vi "写校准时间及fid.vi"(8 "error in (no error)":errorcluster, 9 "量程":u16, 10 "fid":u16, 11 "MB session in":refnum<class "MB_Master.lvclass">) -> (0 "error out":errorcluster, 3 "MB session out":refnum<class "MB_Master.lvclass">)   [LabVIEW 2016, in "MB SLAVE.lvlib"]
uses:
  MB SLAVE.lvlib
  <vilib>/Plasmionique/MB Master/MB_Master/MB_Master.lvclass
  <vilib>/Plasmionique/MB Master/MB Master.lvlib
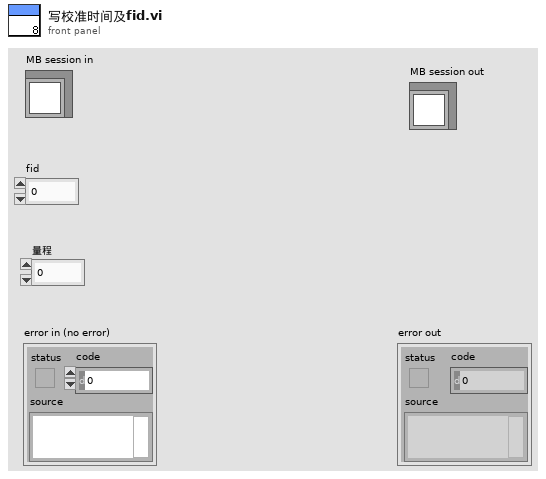
[diagram p1: front panel]
types:
  T1 = typedef "LVDateTimeRec.ctl" = cluster{"秒数的小数部分":dbl, "秒":i32, "分":i32, "时":i32, "日":i32, "月":i32, "年":i32, "天数（周）":i32, "天数（年）":i32, "DST":i32}
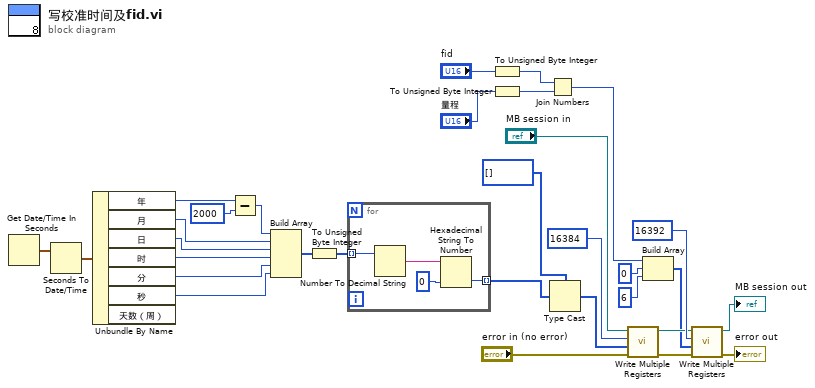
[diagram p0: block diagram]
diagram:
  n1 = Get Date/Time In Seconds() -> (seconds since 1Jan1904=w22:timestamp)
  n2 = Seconds To Date/Time(time stamp (now)=w22) -> (date time rec=w23:T1)  [unwired: 1 in]
  n3 = Unbundle By Name(w23) -> ("年"=w24:i32, "月"=w27:i32, "日"=w28:i32, "时"=w29:i32, "分"=w30:i32, "秒"=w31:i32)  [unwired: 1 out]
  n4 = Subtract(x=w24, y=2000) -> (x-y=w26:i32)
  n5 = Build Array(w26, w27, w28, w29, w30, w31) -> (w2:i32[])
  n6 = To Unsigned Byte Integer(number=w2) -> (unsigned 8bit integer=w4:u8[])
  n7 = for {
    tunnel: w4 -> [w35] mode=indexing
    tunnel: [w32] -> w3 mode=indexing
    n8 = Number To Decimal String(number=w35) -> (decimal integer string=w34:string)  [unwired: 1 in]
    n9 = Hexadecimal String To Number(string=w34, default (0uL)=u8 0 ("默认(0 U32)")) -> (number=w32:u8)  [unwired: 1 in, 1 out]
  }
  n10 = To Unsigned Byte Integer(number="fid") -> (unsigned 8bit integer=w9:u8)
  n11 = To Unsigned Byte Integer(number="量程") -> (unsigned 8bit integer=w8:u8)
  n12 = Join Numbers(hi=w9, lo=w8) -> ((hi.lo)=w7:u16)
  n13 = Type Cast(type=u16[] [], x=w3) -> (*(type *) &x=w1:u16[])
  n14 = call <vilib>:"Write Multiple Registers.vi"("error in (no error)"="error in (no error)", "values"=w1, "starting address"=u16 16384, "MB session in"="MB session in") -> ("error out"=w18:errorcluster, "MB session out"=w19:refnum<class "MB_Master.lvclass">)  [unwired: 6 in]
  n15 = Build Array(w7, u16 0 ("元素"), u16 6 ("元素")) -> (w6:u16[])
  n16 = call <vilib>:"Write Multiple Registers.vi"("error in (no error)"=w18, "values"=w6, "starting address"=u16 16392, "MB session in"=w19) -> ("error out"=→"error out":errorcluster, "MB session out"=→"MB session out":refnum<class "MB_Master.lvclass">)  [unwired: 6 in]
